vi "文本属性.vi"(11 "引用":refnum<vi>) -> ()   [LabVIEW 2020]
panel:
  in  "簇":T1 {"字体" items=["Batang", "Dotum", "方正舒体", "方正姚体", "仿宋", "黑体", "华文彩云", "华文仿宋", "华文楷体", "华文隶书", "华文宋体", "华文细黑", "华文新魏", "华文行楷", "华文中宋", "»ªÎÄçúçê", "楷体", "隶书", "宋体", "微软雅黑", "新宋体", "幼圆"]}
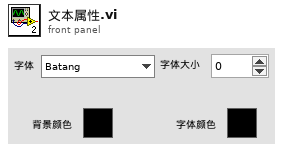
[diagram p1: front panel]
types:
  T1 = cluster{"背景颜色":u32, "字体颜色":u32, "字体":u16, "字体大小":u32}
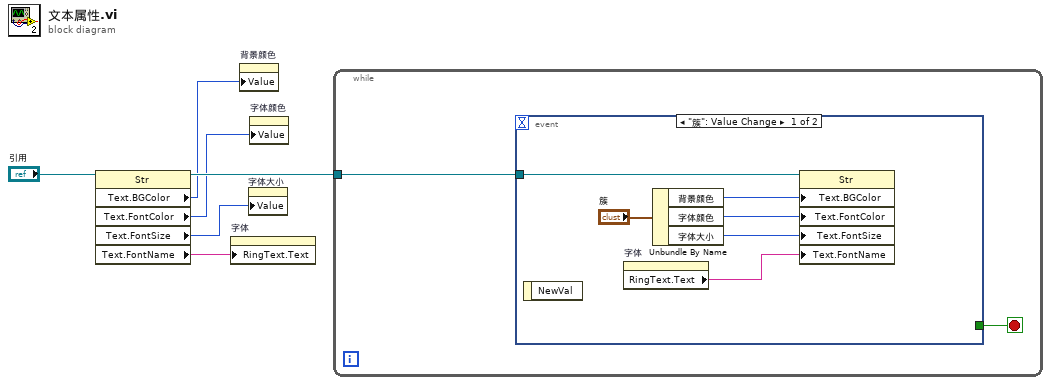
[diagram p0: block diagram]
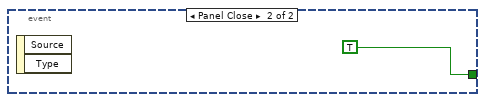
[diagram p2: hidden frame]
diagram:
  n1 = property on="属性节点" class="Str"(reference="引用") -> (reference out=w5:refnum<vi>, "Text.BGColor"=w3:u32, "Text.FontColor"=w2:u32, "Text.FontSize"=w1:u32, "Text.FontName"=w4:string)  [unwired: 1 in, 1 out]
  n2 = property on="字体" class="Ring (strict)"("RingText.Text"=w4) -> ()  [unwired: 2 in, 2 out]
  n3 = property on="背景颜色" class="ColBox"("Value"=w3) -> ()  [unwired: 2 in, 2 out]
  n4 = property on="字体大小" class="DigNum (strict)"("Value"=w1) -> ()  [unwired: 2 in, 2 out]
  n5 = property on="字体颜色" class="ColBox"("Value"=w2) -> ()  [unwired: 2 in, 2 out]
  n6 = while {
    tunnel: w5 -> [w7]
    stop <- w8 stop-if-true
    n7 = event shown="[0] \"簇\": Value Change" {
      selector: _ -> [_ _]
      dyn-events: _ -> [_ _]
      timeout: _ -> [_ _]
      tunnel: w7 -> [w14 _]
      tunnel: [_ TRUE] -> w8
      event "簇": Value Change {
        n8 = event-data() -> ()  [unwired: 1 in, 1 out]
        n9 = property on="字体" class="Ring (strict)"() -> ("RingText.Text"=w9:string)  [unwired: 2 in, 2 out]
        n10 = Unbundle By Name("簇") -> ("背景颜色"=w12:u32, "字体颜色"=w11:u32, "字体大小"=w10:u32)
        n11 = property on="属性节点" class="Str"(reference=w14, "Text.BGColor"=w12, "Text.FontColor"=w11, "Text.FontSize"=w10, "Text.FontName"=w9) -> ()  [unwired: 1 in, 2 out]
      }
      event Panel Close {
        n12 = event-data() -> ()  [unwired: 1 in, 2 out]
      }
    }
  }
